vi "varToRobcomm.vi"(1 "var name":string, 2 "var value":dbl=9.5, 3 "VISA resource name":refnum<visa-resource-name>) -> (0 "VISA resource name out":refnum<visa-resource-name>)   [LabVIEW 2012]
panel:
  out "return count":u32
  out "concatenated string":string
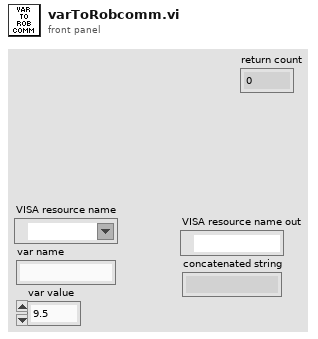
[diagram p1: front panel]
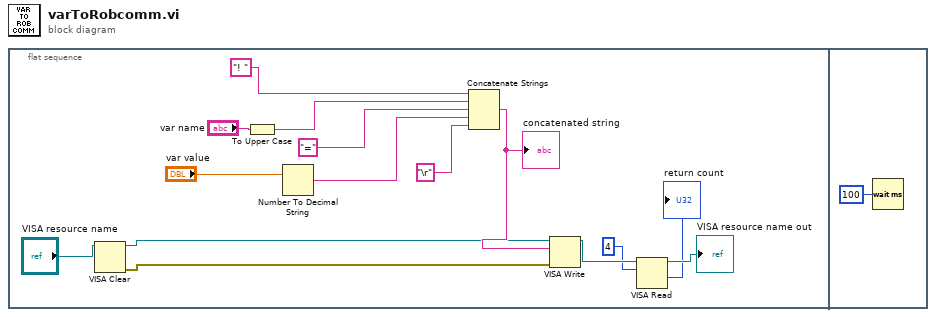
[diagram p0: block diagram]
diagram:
  n1 = flat-sequence {
    frame #0 {
      n2 = VISA Clear(VISA resource name="VISA resource name") -> (VISA resource name out=w7:refnum<visa-resource-name>, error out=w6:errorcluster)  [unwired: 1 in]
      n3 = To Upper Case(1:"var name") -> (0:w9:string)
      n4 = Number To Decimal String(number="var value") -> (decimal integer string=w13:string)  [unwired: 1 in]
      n5 = Concatenate Strings("! " ("write buffer"), w9, "=" ("write buffer"), w13, "\r" ("string")) -> (w15:string)
      "concatenated string" <- w15
      n6 = VISA Write(VISA resource name=w7, write buffer=w15, error in (no error)=w6) -> (VISA resource name out=w4:refnum<visa-resource-name>)  [unwired: 2 out]
      n7 = VISA Read(VISA resource name=w4, byte count=u32 4) -> (VISA resource name out=→"VISA resource name out":refnum<visa-resource-name>, return count=→"return count":u32)  [unwired: 1 in, 2 out]
    }
    frame #1 {
      n8 = Wait (ms)(milliseconds to wait=u32 100) -> ()  [unwired: 1 out]
    }
  }
